vi "Read_101.vi"(0 "Modbus instance in":refnum<class "Modbus API.lvclass">, 11 "error in (no error)":errorcluster) -> (4 "Modbus instance out":refnum<class "Modbus API.lvclass">, 6 "Р пластовое":sgl format="%#.3f", 8 "Р горное":sgl format="%#.3f", 10 "Р атм.":sgl format="%#.4f", 13 "Температура":sgl format="%#.4f", 15 "error out":errorcluster)   [LabVIEW 2018]
uses:
  <vilib>/NI/Modbus Library/API/Modbus API.lvclass
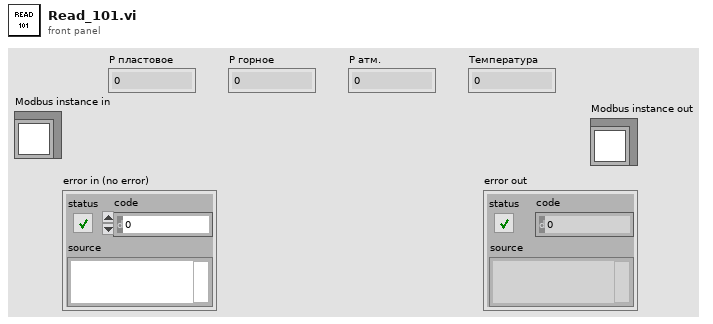
[diagram p1: front panel]
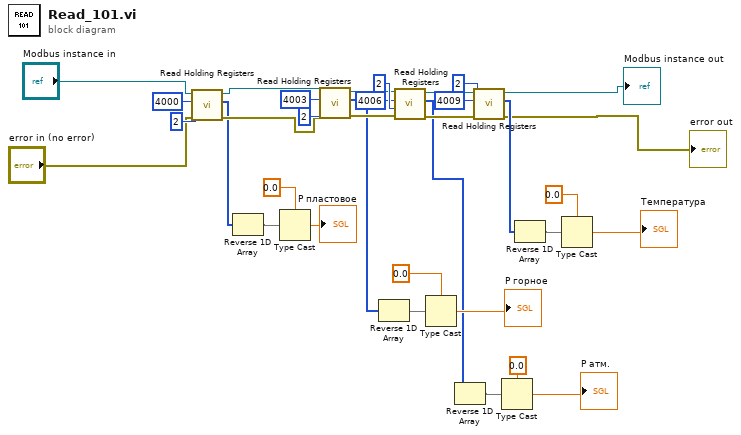
[diagram p0: block diagram]
diagram:
  n1 = call-dynamic "Read Holding Registers.vi"("error in"="error in (no error)", "number of inputs"=u16 2, "starting address"=u16 4000, "Modbus instance in"="Modbus instance in") -> ("error out"=w12:errorcluster, "register values"=w8:u16[], "Modbus instance out"=w11:refnum<class "Modbus API.lvclass">)  [unwired: 5 in]
  n2 = Reverse 1D Array(array=w8) -> (reversed array=w15:u16[])
  n3 = Type Cast(type=sgl 0.0, x=w15) -> (*(type *) &x=→"Р пластовое":sgl)
  n4 = call-dynamic "Read Holding Registers.vi"("error in"=w12, "number of inputs"=u16 2, "starting address"=u16 4003, "Modbus instance in"=w11) -> ("error out"=w27:errorcluster, "register values"=w7:u16[], "Modbus instance out"=w28:refnum<class "Modbus API.lvclass">)  [unwired: 5 in]
  n5 = Reverse 1D Array(array=w7) -> (reversed array=w24:u16[])
  n6 = call-dynamic "Read Holding Registers.vi"("error in"=w27, "number of inputs"=u16 2, "starting address"=u16 4006, "Modbus instance in"=w28) -> ("error out"=w31:errorcluster, "register values"=w6:u16[], "Modbus instance out"=w32:refnum<class "Modbus API.lvclass">)  [unwired: 5 in]
  n7 = Type Cast(type=sgl 0.0, x=w24) -> (*(type *) &x=→"Р горное":sgl)
  n8 = Reverse 1D Array(array=w6) -> (reversed array=w20:u16[])
  n9 = call-dynamic "Read Holding Registers.vi"("error in"=w31, "number of inputs"=u16 2, "starting address"=u16 4009, "Modbus instance in"=w32) -> ("error out"=→"error out":errorcluster, "register values"=w5:u16[], "Modbus instance out"=→"Modbus instance out":refnum<class "Modbus API.lvclass">)  [unwired: 5 in]
  n10 = Type Cast(type=sgl 0.0, x=w20) -> (*(type *) &x=→"Р атм.":sgl)
  n11 = Reverse 1D Array(array=w5) -> (reversed array=w23:u16[])
  n12 = Type Cast(type=sgl 0.0, x=w23) -> (*(type *) &x=→"Температура":sgl)
